vi "Connection MySQL.vi"() -> ()   [LabVIEW 2021]
uses:
  <vilib>/addons/database/Connection.llb/DB Tools Open Connec (String).vi
  <vilib>/addons/database/NI_Database_API.lvlib
  <vilib>/addons/database/Connection.llb/DB Tools Open Connec (Path).vi
panel:
  out "error out":errorcluster
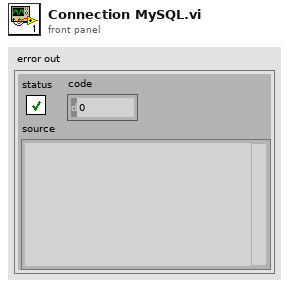
[diagram p1: front panel]
types:
  T1 = typedef "NI_Database_API.lvlib/Conn ObjectReference.ctl" = refnum<k1>
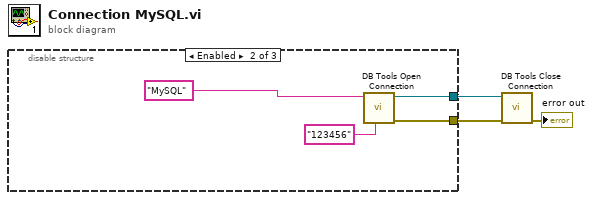
[diagram p0: block diagram]
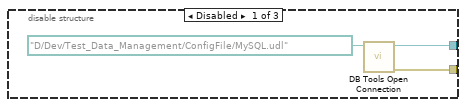
[diagram p2: hidden frame]
diagram:
  n1 = disable-structure shown="Enabled" {
    disable-tunnel: [w5 w10 _] -> w3
    disable-tunnel: [w4 w9 _] -> w2
    frame Disabled {
      n2 = call-poly <vilib>:"DB Tools Open Connection.vi"("connection information"=path "D:/Dev/Test_Data_Management/ConfigFile/MySQL.udl") -> ("error out"=w4:errorcluster, "connection reference"=w5:T1)  [unwired: 7 in]
    }
    frame Enabled {
      n3 = call-poly <vilib>:"DB Tools Open Connection.vi"("password"="123456", "connection information"="MySQL" ("userID")) -> ("error out"=w9:errorcluster, "connection reference"=w10:T1)  [unwired: 6 in]
    }
    frame Disabled {
    }
  }
  n4 = call <vilib>:"DB Tools Close Connection.vi"("error in (no error)"=w2, "connection reference"=w3) -> ("error out"=→"error out":errorcluster)  [unwired: 5 in]
